vi "Snap to Heading.vi"(8 "Rotational - Z":dbl, 11 "Lateral - X":dbl) -> (3 "Rotational - Z":dbl format="%.2f")   [LabVIEW 2018]
uses:
  <vilib>/addons/control/pid/pid.llb/PID (DBL).vi
  <vilib>/addons/control/pid/NI_PID_pid.lvlib
panel:
  out "PID Output":dbl format="%.2f"
  out "Yaw Setpoint":dbl
  out "Connected":bool
  out "YRPHfH":T1
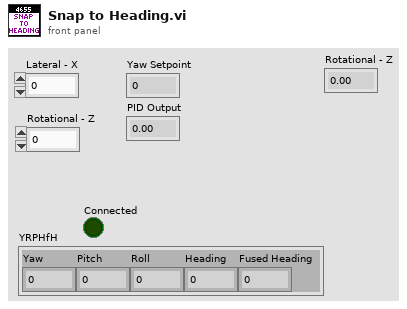
[diagram p1: front panel]
types:
  T1 = cluster{"Yaw":dbl, "Pitch":dbl, "Roll":dbl, "Heading":dbl, "Fused Heading":dbl}
  T2 = cluster{"proportional gain (Kc)":dbl, "integral time (Ti, min)":dbl, "derivative time (Td, min)":dbl}
  T3 = cluster{"Yaw":dbl, "Roll":dbl, "Pitch":dbl, "Heading":dbl, "Fused Heading":dbl}
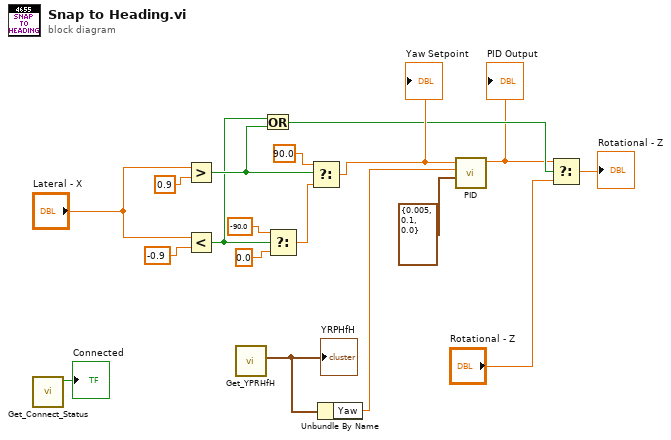
[diagram p0: block diagram]
diagram:
  n1 = call <vilib>:"Get_Connect_Status.vi"() -> ("Connected"=→"Connected":bool)  [unwired: 11 in]
  n2 = Greater?(x="Lateral - X", y=0.9) -> (0:w9:bool)
  n3 = Less?(x="Lateral - X", y=-0.9) -> (x < y?=w8:bool)
  n4 = call <vilib>:"Get_YPRHfH.vi"() -> ("YRPHfH"=w18:T3)  [unwired: 11 in]
  "YRPHfH" <- w18
  n5 = Or(x=w8, y=w9) -> (x .or. y?=w5:bool)
  n6 = Select(t=-90.0, s=w8, f=0.0) -> (s? t:f=w12:dbl)
  n7 = Select(t=90.0, s=w9, f=w12) -> (s? t:f=w7:dbl)
  "Yaw Setpoint" <- w7
  n8 = Unbundle By Name(w18) -> ("Yaw"=w6:dbl)
  n9 = call-poly <vilib>:"PID.vi"("PID gains"=T2 {"proportional gain (Kc)"=0.005, "integral time (Ti, min)"=0.1, "derivative time (Td, min)"=0.0}, "process variable"=w6, "setpoint"=w7) -> ("output"=w4:dbl)  [unwired: 7 in, 1 out]
  "PID Output" <- w4
  n10 = Select(t=w4, s=w5, f="Rotational - Z") -> (s? t:f=→"Rotational - Z":dbl)
